vi "status_loop.vi"(8 "error in (no error)":errorcluster) -> (0 "error out":errorcluster)   [LabVIEW 2012]
uses:
  <vilib>/Platform/TimedLoop/XDataNode/timing_clust.ctl
  <vilib>/Platform/TimedLoop/XDataNode/nitl_modes.ctl
  <vilib>/Platform/TimedLoop/XDataNode/wakeup.ctl
  initialization/micron_globals.vi
  <vilib>/Platform/TimedLoop/XDataNode/XDataNode.xnode
  <vilib>/Platform/TimedLoop/XDataNode/XDNodeRunTimeDep.lvlib
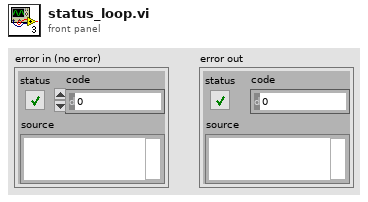
[diagram p1: front panel]
types:
  T1 = typedef "XDNodeRunTimeDep.lvlib/timing_clust.ctl" = cluster{"Expected End [f-1]":u64, "Actual End [f-1]":u64, "Finished Late? [f-1]":bool, "Expected End [i-1]":u64, "Actual End [i-1]":u64, "Finished Late? [i-1]":bool, "Expected Start [i]":u64, "Actual Start [i]":u64, "Expected Start [f]":u64, "Actual Start [f]":u64, "Source Name":string, "Structure Name":string, "Period":i64, "Deadline":i64, "Offset":i64, "Start":i64, "Priority":i32, "Timeout":i32, "Mode":T2, "Wakeup Reason":T3, "Error":errorcluster, "Source Type":string, "Secondary Source Type":string, "Global End Time":u64, "Global Start Time":u64, "Frame Duration":u64, "Iteration Duration":u64, "Assigned CPU":i32, "I/O Scan Engine Mode":u32}
  T2 = typedef "XDNodeRunTimeDep.lvlib/nitl_modes.ctl" = enum32{"No Change", "Process missed periods, maintain original phase", "Discard missed periods, maintain original phase", "Process missed periods, ignore original phase", "Discard missed periods, ignore original phase"}
  T3 = typedef "XDNodeRunTimeDep.lvlib/wakeup.ctl" = enum32{"Normal", "Aborted", "Asynchronous wakeup", "Timing source error", "Timed loop error", "Timeout"}
  T4 = typedef "log_event.ctl" = cluster{"Facility ID":i32, "Severity":enum16{"OK", "Debug", "Warn", "Error"}, "Timestamp":timestamp, "Facility":string, "State":string, "Message":string}
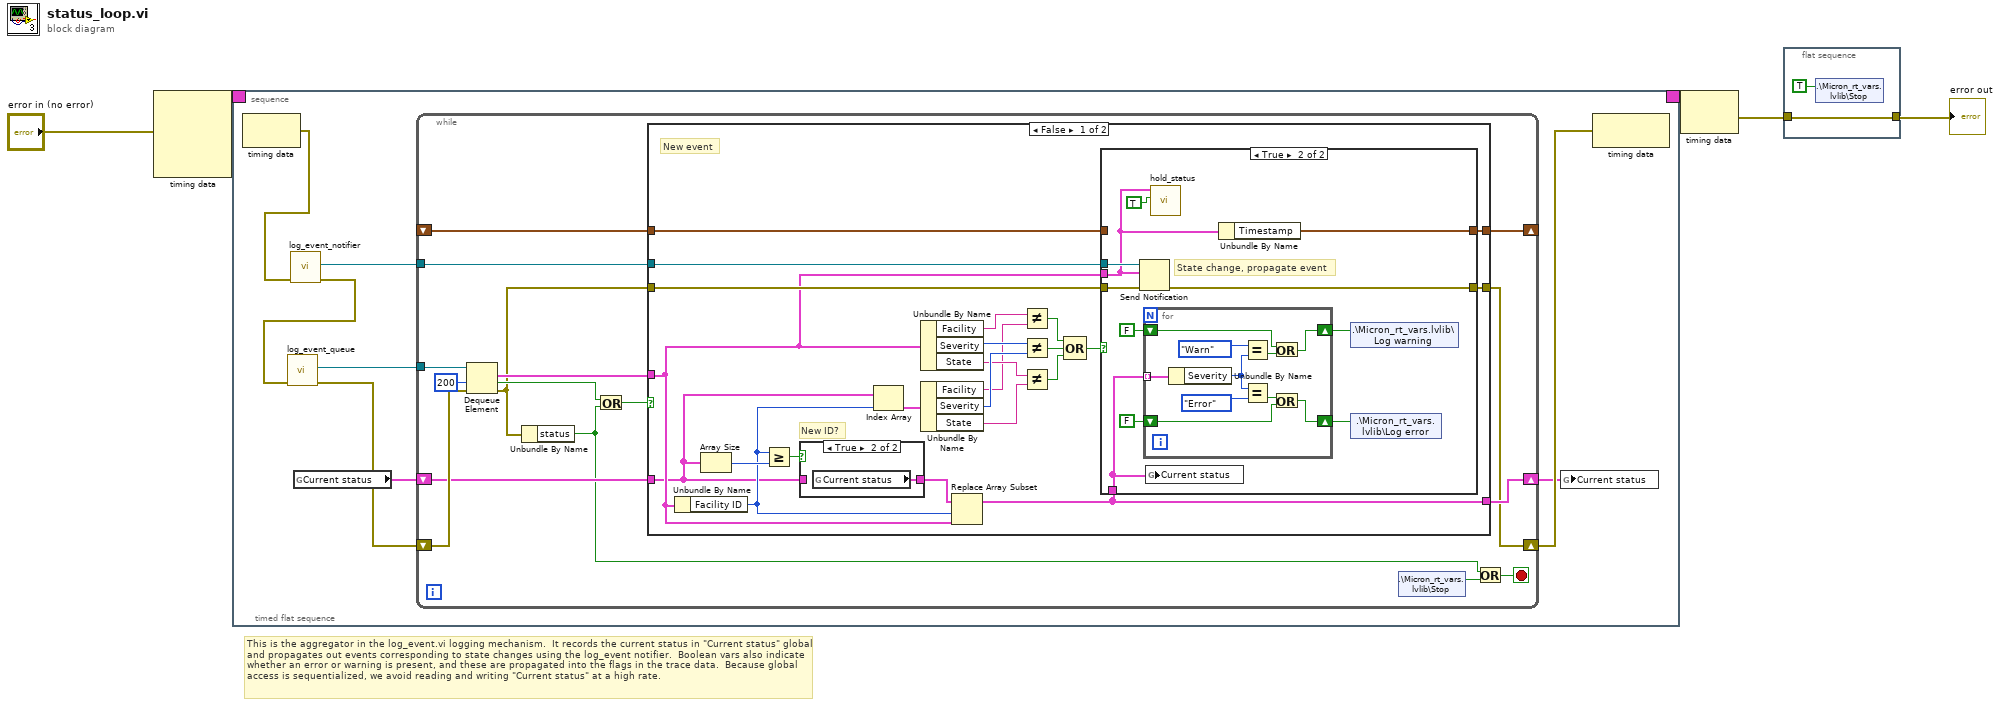
[diagram p0: block diagram]
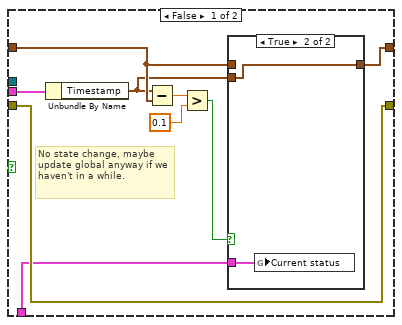
[diagram p3: hidden frame]
diagram:
  # "This is the aggregator in the log_event.vi logging mechanism.  It records the current status in \"Current status\" global and propagates out events corresponding to state changes using the log_event notifier.  Boolean vars also indicate whether an error or warning is present, and these are propagated into the flags in the trace data.  Because global access is sequentialized, we avoid reading and writing \"Current status\" at a high rate."
  n1 = node-c288("error in (no error)") -> (w5:T1)  [unwired: 3 in]
  n2 = timed-sequence {
    timing: w5 -> [_]
    timing-out: [_] -> w4
    n3 = timed-flat-sequence {
      n4 = node-c288() -> (w6:errorcluster)  [unwired: 1 in]
      n5 = call "log_event_notifier.vi"("error in"=w6) -> ("error out"=w8:errorcluster, "Log event notifier"=w7:refnum<notifier>)  [unwired: 9 in]
      n6 = call "log_event_queue.vi"("error in"=w8) -> ("error out"=w12:errorcluster, "Log event queue"=w13:refnum<queue>)  [unwired: 9 in]
      n7 = global read "micron_globals.vi" "Current status"() -> (w11:T4[])
      n8 = while {
        tunnel: w13 -> [w29]
        shift-right: [w24] -> w9
        shift-left: w11 -> [w25]
        tunnel: w7 -> [w18]
        shift-right: [w16] -> w10
        shift-left: w12 -> [w28]
        shift-right: [w15] -> _
        shift-left: _ -> [w14]
        stop <- w23 stop-if-true
        n9 = Dequeue Element(queue=w29, timeout in ms (-1)=200, error in (no error)=w28) -> (element=w26:T4, timed out?=w20:bool, error out=w17:errorcluster)  [unwired: 1 out]
        n10 = Unbundle By Name(w17) -> ("status"=w19:bool)
        n11 = Or(x=w20, y=w19) -> (x .or. y?=w21:bool)
        n12 = case shown="False" w21 {
          tunnel: w26 -> [w37 _]
          tunnel: w25 -> [w30 w90]
          tunnel: [w44 w90] -> w24
          tunnel: w18 -> [w41 _]
          tunnel: w17 -> [w40 w89]
          tunnel: [w39 w89] -> w16
          tunnel: [w36 w88] -> w15
          tunnel: w14 -> [w35 w88]
          frame False {
            # "New ID?"
            # "New event"
            n13 = Unbundle By Name(w37) -> ("Facility ID"=w33:i32)
            n14 = Array Size(array=w30) -> (size(s)=w34:i32)
            n15 = Greater Or Equal?(x=w33, y=w34) -> (x >= y?=w32:bool)
            n16 = case shown="True" w32 {
              tunnel: [w53 w54] -> w31
              tunnel: w30 -> [w53 _]
              frame False {
              }
              frame True {
                n17 = global read "micron_globals.vi" "Current status"() -> (w54:T4[])
              }
            }
            n18 = Index Array(array=w30, index=w33) -> (element=w52:T4)
            n19 = Unbundle By Name(w37) -> ("Facility"=w43:string, "Severity"=w51:enum16{"OK", "Debug", "Warn", "Error"}, "State"=w49:string)
            n20 = Unbundle By Name(w52) -> ("Facility"=w38:string, "Severity"=w50:enum16{"OK", "Debug", "Warn", "Error"}, "State"=w48:string)
            n21 = Replace Array Subset(array=w31, new element=w37, index=w33) -> (w44:T4[])
            n22 = Not Equal?(x=w43, y=w38) -> (x != y?=w42:bool)
            n23 = Not Equal?(x=w51, y=w50) -> (x != y?=w47:bool)
            n24 = Not Equal?(x=w49, y=w48) -> (x != y?=w46:bool)
            n25 = Compound Arithmetic op=OR(w42, w47, w46) -> (w45:bool)
            n26 = case shown="True" w45 {
              tunnel: w44 -> [w59 w74]
              tunnel: w41 -> [_ w77]
              tunnel: w40 -> [w61 w76]
              tunnel: [w61 w75] -> w39
              tunnel: w37 -> [w63 w68]
              tunnel: [w56 w69] -> w36
              tunnel: w35 -> [w57 _]
              frame False {
                # "No state change, maybe update global anyway if we haven't in a while."
                n27 = Unbundle By Name(w63) -> ("Timestamp"=w55:timestamp)
                n28 = Subtract(x=w55, y=w57) -> (x-y=w62:dbl)
                n29 = Greater?(x=w62, y=0.1) -> (0:w58:bool)
                n30 = case shown="True" w58 {
                  tunnel: w59 -> [_ w66]
                  tunnel: w57 -> [w64 _]
                  tunnel: [w64 w65] -> w56
                  tunnel: w55 -> [_ w65]
                  frame False {
                  }
                  frame True {
                    n31 = global write "micron_globals.vi" "Current status"(w66) -> ()
                  }
                }
              }
              frame True {
                # "State change, propagate event"
                n32 = Send Notification(notification=w68, notifier=w77, error in (no error)=w76) -> (error out=w75:errorcluster)  [unwired: 1 out]
                n33 = for {
                  tunnel: w74 -> [w87] mode=indexing
                  shift-right: [w84] -> w71
                  shift-left: FALSE -> [w83]
                  shift-right: [w79] -> w70
                  shift-left: FALSE -> [w78]
                  n34 = Unbundle By Name(w87) -> ("Severity"=w80:enum16{"OK", "Debug", "Warn", "Error"})
                  n35 = Equal?(x=enum16{"OK", "Debug", "Warn", "Error"}."Warn", y=w80) -> (x = y?=w85:bool)
                  n36 = Equal?(x=w80, y=enum16{"OK", "Debug", "Warn", "Error"}."Error" ("x")) -> (x = y?=w82:bool)
                  n37 = Or(x=w83, y=w85) -> (x .or. y?=w84:bool)
                  n38 = Or(x=w82, y=w78) -> (x .or. y?=w79:bool)
                }
                n39 = global write "micron_globals.vi" "Current status"(w74) -> ()
                n40 = call "hold_status.vi"("Update"=TRUE, "New event"=w68) -> ()  [unwired: 7 in, 3 out]
                n41 = Unbundle By Name(w68) -> ("Timestamp"=w69:timestamp)
                n42 = shared-variable ".\\Micron_rt_vars.lvlib\\Log warning"(w71) -> ()  [unwired: 1 in, 1 out]
                n43 = shared-variable ".\\Micron_rt_vars.lvlib\\Log error"(w70) -> ()  [unwired: 1 in, 1 out]
              }
            }
          }
          frame True {
            # "Timeout, no recent events.  This isn't likely to happen unless state updates are quite slow."
          }
        }
        n44 = shared-variable ".\\Micron_rt_vars.lvlib\\Stop"() -> (w22:bool)  [unwired: 2 out]
        n45 = Or(x=w19, y=w22) -> (x .or. y?=w23:bool)
      }
      n46 = global write "micron_globals.vi" "Current status"(w9) -> ()
      n47 = node-c288(w10) -> ()  [unwired: 1 out]
    }
  }
  n48 = node-c288(w4) -> (w2:errorcluster)
  n49 = flat-sequence {
    tunnel: w2 -> [w96]
    tunnel: [w96] -> w1
    frame #0 {
      n50 = shared-variable ".\\Micron_rt_vars.lvlib\\Stop"(TRUE ("Stop")) -> ()  [unwired: 2 out]
    }
  }
  "error out" <- w1
